vi "remove missing channels.vi"(8 "error in":errorcluster, 10 "module configurations":refnum<class "TBM module configuration.lvclass">[](array[class]), 11 "engine configuration in":refnum<class "engine configuration.lvclass">) -> (0 "error out":errorcluster, 3 "engine configuration out":refnum<class "engine configuration.lvclass">)   [LabVIEW 2013, in "engine configuration.lvclass"]
doc: "This function checks the list of mapped channels that the engine configuration is aware of based on the identifier of the module and removes any channels that the module no longer claims to contain. This function is used to synchronize the engine configuration with the configurations of the modules that were input."
uses:
  engine configuration.lvclass
  <vilib>/NI/Tag Bus Module Framework/module configuration/TBM module configuration.lvclass
  <vilib>/NI/Configuration Framework/serializable configuration/NISE_CEF_serializable configuration.lvclass/NISE_CEF_serializable configuration.ctl
  <vilib>/NI/Tag Bus/tag/tag descriptor.lvclass/tag descriptor.ctl
  <vilib>/NI/Tag Bus Module Framework/channel/TBM channel.lvclass/TBM channel.ctl
  <vilib>/NI/Tag Bus/tag/read data type.vi
  <vilib>/NI/Tag Bus Module Framework/channel/Read channel classification.vi
  <vilib>/NI/Tag Bus/tag/read tag name.vi
  <vilib>/Utility/LVClass/Get LV Class Name.vi
  <vilib>/NI/Configuration Framework/error generator.vi
  <vilib>/NI/Tag Bus/tag/tag descriptor.lvclass
  <vilib>/NI/Tag Bus Module Framework/channel/TBM channel.lvclass
  <vilib>/NI/Configuration Framework/serializable configuration/NISE_CEF_serializable configuration.lvclass
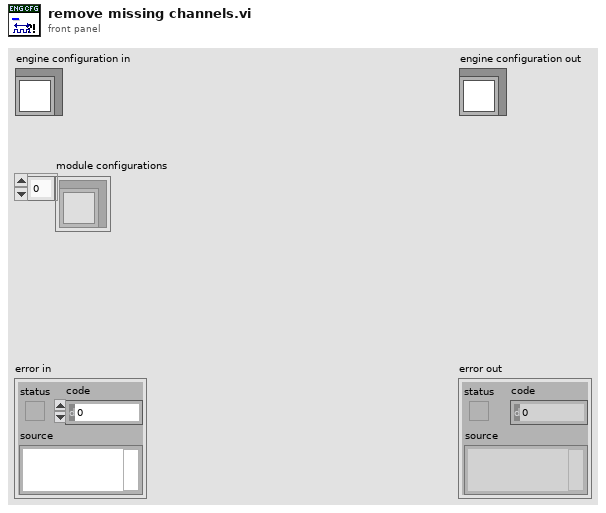
[diagram p1: front panel]
types:
  T1 = typedef "tag bus.lvlib/tag descriptor.lvclass/Data Type.ctl" = enum16{"Double", "Single", "I64", "I32", "I16", "I8", "U64", "U32", "U16", "U8", "Boolean", "String", "Array of Double", "Array of Single", "Array of I64", "Array of I32", "Array of I16", "Array of I8", "Array of U64", "Array of U32", "Array of U16", "Array of U8", "Array of Boolean", "Array of String"}
  T2 = typedef "TBM channel.lvclass/channel classification.ctl" = enum16{"input data", "output data", "processing parameter", "processing result"}
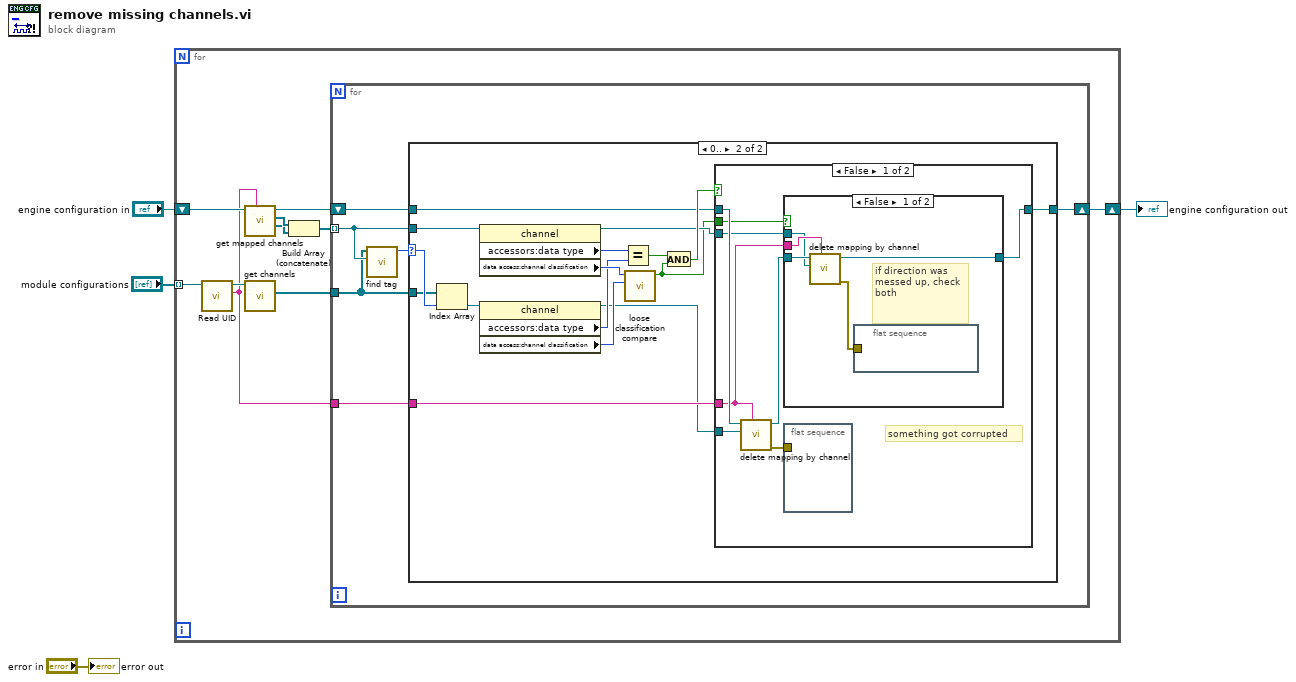
[diagram p0: block diagram]
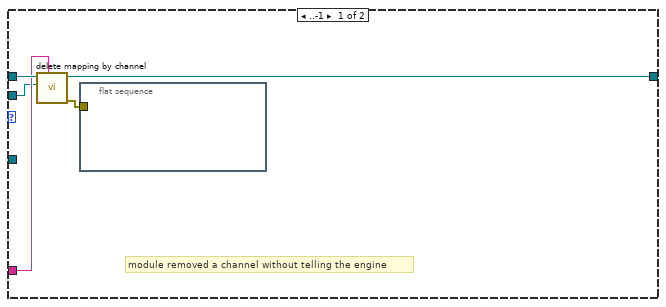
[diagram p2: hidden frame]
diagram:
  n1 = for {
    tunnel: "module configurations" -> [w14] mode=indexing
    shift-right: [w10] -> w2
    shift-left: "engine configuration in" -> [w12]
    n2 = call <vilib>:"Read UID.vi"("configuration in"=w14) -> ("instance id"=w5:string, "configuration out"=w13:refnum<class "TBM module configuration.lvclass">)  [unwired: 8 in, 1 out]
    n3 = call "get mapped channels.vi"("owner"=w5, "engine configuration in"=w12) -> ("write channels"=w7:refnum<class "TBM channel.lvclass">[], "read channels"=w8:refnum<class "TBM channel.lvclass">[], "engine configuration out"=w11:refnum<class "engine configuration.lvclass">)  [unwired: 5 in, 2 out]
    n4 = call-dynamic "get channels.vi"("module configuration in"=w13) -> ("channels"=w9:refnum<class "TBM channel.lvclass">[])  [unwired: 9 in, 1 out]
    n5 = Build Array (concatenate)(w8, w7) -> (w6:refnum<class "TBM channel.lvclass">[])
    n6 = for {
      shift-right: [w17] -> w10
      shift-left: w11 -> [w19]
      tunnel: w9 -> [w15]
      tunnel: w6 -> [w16] mode=indexing
      tunnel: w5 -> [w18]
      n7 = call <vilib>:"find tag.vi"("tag"=w16, "tags in"=w15) -> ("index"=w20:i32)  [unwired: 9 in]
      n8 = case shown="0.." w20 {
        selector: w20 -> [_ w41]
        tunnel: w19 -> [w25 w30]
        tunnel: w18 -> [w23 w29]
        tunnel: [w24 w31] -> w17
        tunnel: w16 -> [w21 w38]
        tunnel: w15 -> [_ w40]
        frame ..-1 {
          # "module removed a channel without telling the engine"
          n9 = call "delete mapping by channel.vi"("owner ID"=w23, "channel"=w21, "engine configuration in"=w25) -> ("error out"=w22:errorcluster, "engine configuration out"=w24:refnum<class "engine configuration.lvclass">)  [unwired: 7 in]
          n10 = flat-sequence {
            tunnel: w22 -> [_]
            frame #0 {
            }
          }
        }
        frame 0.. {
          n11 = Index Array(array=w40, index=w41) -> (element=w39:refnum<class "TBM channel.lvclass">)
          n12 = property class="channel"(reference=w38) -> (reference out=w27:refnum<class "TBM channel.lvclass">, "accessors:data type"=w35:T1, "data access:channel classification"=w37:T2)  [unwired: 1 in, 1 out]
          n13 = property class="channel"(reference=w39) -> (reference out=w28:refnum<class "TBM channel.lvclass">, "accessors:data type"=w34:T1, "data access:channel classification"=w36:T2)  [unwired: 1 in, 1 out]
          n14 = Equal?(x=w35, y=w34) -> (x = y?=w33:bool)
          n15 = call "loose classification compare.vi"("class 2"=w36, "class 1"=w37) -> ("match?"=w26:bool)  [unwired: 9 in]
          n16 = And(x=w33, y=w26) -> (x .and. y?=w32:bool)
          n17 = case shown="False" w32 {
            tunnel: [w45 w56] -> w31
            tunnel: w30 -> [w48 w56]
            tunnel: w29 -> [w44 _]
            tunnel: w28 -> [w47 _]
            tunnel: w27 -> [w43 _]
            tunnel: w26 -> [w42 _]
            frame False {
              # "something got corrupted"
              n18 = call "delete mapping by channel.vi"("owner ID"=w44, "channel"=w47, "engine configuration in"=w48) -> ("error out"=w49:errorcluster, "engine configuration out"=w46:refnum<class "engine configuration.lvclass">)  [unwired: 7 in]
              n19 = case shown="False" w42 {
                tunnel: w46 -> [w54 w55]
                tunnel: [w53 w55] -> w45
                tunnel: w44 -> [w51 _]
                tunnel: w43 -> [w50 _]
                frame False {
                  # "if direction was messed up, check both"
                  n20 = call "delete mapping by channel.vi"("owner ID"=w51, "channel"=w50, "engine configuration in"=w54) -> ("error out"=w52:errorcluster, "engine configuration out"=w53:refnum<class "engine configuration.lvclass">)  [unwired: 7 in]
                  n21 = flat-sequence {
                    tunnel: w52 -> [_]
                    frame #0 {
                    }
                  }
                }
                frame True {
                }
              }
              n22 = flat-sequence {
                tunnel: w49 -> [_]
                frame #0 {
                }
              }
            }
            frame True {
              # "ok"
            }
          }
        }
      }
    }
  }
  "engine configuration out" <- w2
  "error out" <- "error in"
